vi "Reinterpret U16 as I16.vi"(7 "Input":u16) -> (8 "Output":i16)   [LabVIEW 2012]
uses:
  <vilib>/rvi/FXPMathLib/FxpInterpret/XNode/nifxpmath_Interpret.xnode
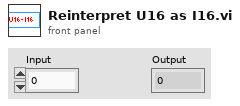
[diagram p1: front panel]
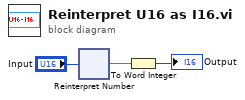
[diagram p0: block diagram]
diagram:
  n1 = xnode "Reinterpret Number"("x"="Input") -> ("y"=w3:fxp<+/-,16,16>)
  n2 = To Word Integer(number=w3) -> (16bit integer=→"Output":i16)
